vi "Get Monkey ID From FPGA Name.vi"(8 "error in (no error)":errorcluster, 10 "FPGA Name":string, 11 "Tamer in":refnum<class "Tamer.lvclass">) -> (0 "error out":errorcluster, 2 "Monkey ID":string, 3 "Tamer out":refnum<class "Tamer.lvclass">)   [LabVIEW 2020, in "Tamer.lvlib" / "Tamer.lvclass"]
uses:
  Tamer.lvclass
  Tamer.lvclass/Tamer.ctl
  TALOS/TALOS_PPL.lvlibp
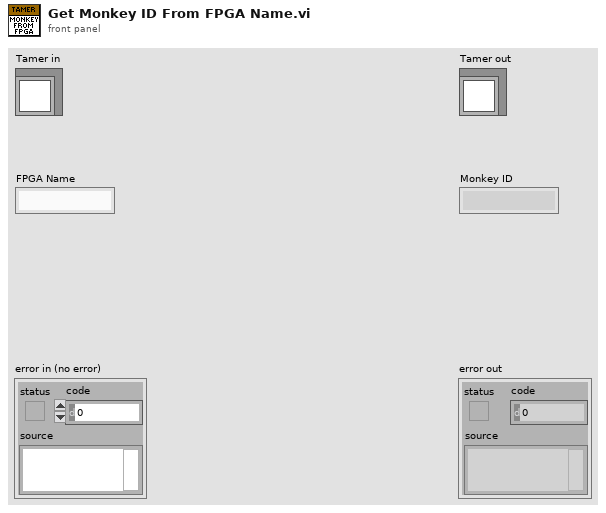
[diagram p1: front panel]
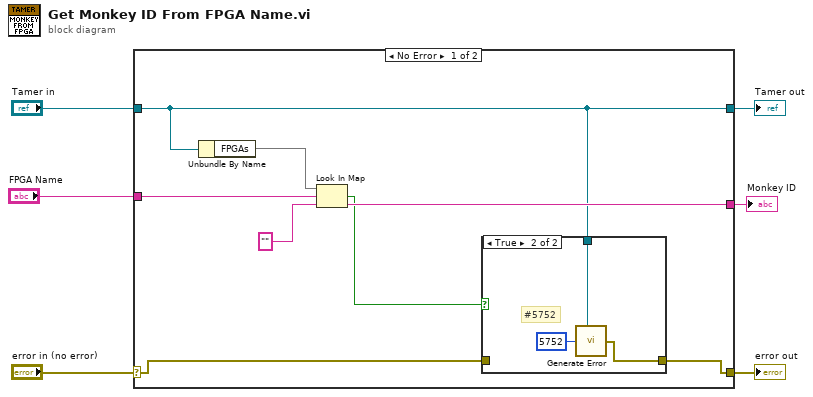
[diagram p0: block diagram]
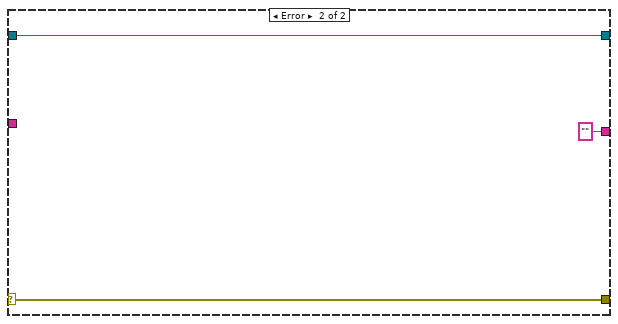
[diagram p3: hidden frame]
diagram:
  n1 = case shown="No Error" "error in (no error)" {
    selector: "error in (no error)" -> [w9 w21]
    tunnel: [w8 w21] -> w5
    tunnel: [w7 w20] -> w3
    tunnel: "Tamer in" -> [w7 w20]
    tunnel: "FPGA Name" -> [w13 _]
    tunnel: [w11 "" ("Monkey uService")] -> w1
    frame No Error {
      n2 = Unbundle By Name(w7) -> ("FPGAs"=w14:map{string, string})
      n3 = Look In Map(map=w14, key=w13, default value="") -> (key not found?=w10:bool, value=w11:string)
      n4 = case shown="True" w10 {
        tunnel: w9 -> [w15 _]
        tunnel: [w15 w17] -> w8
        tunnel: w7 -> [_ w18]
        frame False {
        }
        frame True {
          # "#5752"
          n5 = call "Generate Error.vi"("Class"=w18, "Error Code"=5752) -> ("error out"=w17:errorcluster)  [unwired: 5 in]
        }
      }
    }
    frame Error {
    }
  }
  "error out" <- w5
  "Tamer out" <- w3
  "Monkey ID" <- w1
